vi "BIN-date2weekNum.vi"(2 "Time":timestamp) -> (7 "WeekNum":u64)   [LabVIEW 2020, in "Sgraph_lib_V1.lvlib" / "DBAL-BIN.lvclass"]
doc: "Convert date to West European Weak numerical value"
uses:
  DBAL-BIN.lvclass
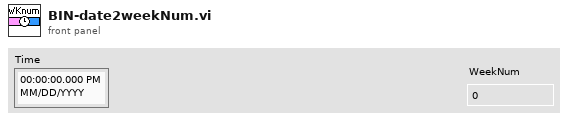
[diagram p1: front panel]
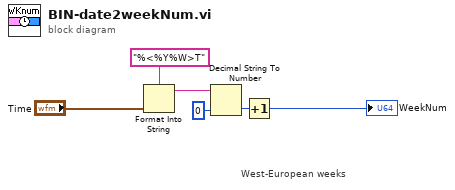
[diagram p0: block diagram]
diagram:
  # "West-European weeks"
  n1 = Format Into String(format string="%<%Y%W>T", "Time") -> (resulting string=w5:string)  [unwired: 2 in, 1 out]
  n2 = Decimal String To Number(string=w5, default (0L)=u64 0 ("default (0 I32)")) -> (number=w4:u64)  [unwired: 1 in, 1 out]
  n3 = Increment(x=w4) -> (x+1=→"WeekNum":u64)
